vi "DiffDriveTrainSim_GetOutput_Single.vi"(9 "Row":i32, 11 "DiffDriveTrainSim":T1 {"m_Motor"."Jr_KgM2" format="%13.5p"; "m_Motor"."L_H" format="%13.5p"; "m_Motor"."Kt_NMPerAmp" format="%13.5p"; "m_Motor"."KvINV_RadPerSecPerVolt" format="%13.5p"; "m_Motor"."R_Ohms" format="%13.5p"; "m_Motor"."FreeSpeed_RadPerSec" format="%13.5p"; "m_Motor"."FreeCurrent_Amps" format="%13.5p"; "m_Motor"."StallCurrent_Amps" format="%13.5p"; "m_Motor"."StallTorque_NM" format="%13.5p"; "m_Motor"."nominalVoltage_Volts" format="%13.5p"}) -> (3 "Output":dbl)   [LabVIEW 2019, in "Trajectory_Library.lvlib"]
doc: "Get the output \n\nInputs:\n - DiffDriveTraimSim -- Data cluster\n - Row -- The desired row.\n values correspond to:\n 0 = X\n 1 = Y\n 2 = Heading\n 3 = LeftVelocity\n 4 = RightVelocity\n 5 = LeftPosition\n 6 = RightPosition\n\nOutputs:\n - Output -- The output value"
uses:
  Trajectory_Library.lvlib
  TypeDef/LINEAR_SYSTEM.ctl
  <vilib>/Analysis/Matrix/Datatypes/RealMatrix.ctl
  <vilib>/Analysis/Matrix/NI_Matrix.lvlib
  TypeDef/DCMOTOR.CTL
  TypeDef/DIFF_DRIVE_TRAIN_SIM.ctl
panel:
  # "<States, 1>"
  # "<Outputs, 1>"
  # "<Inputs, 1>"
  # "<Outputs, 1>"
  # "<States,States>"
  # "<States,Inputs>"
  # "<Outputs,States>"
  # "<Outputs,Inputs>"
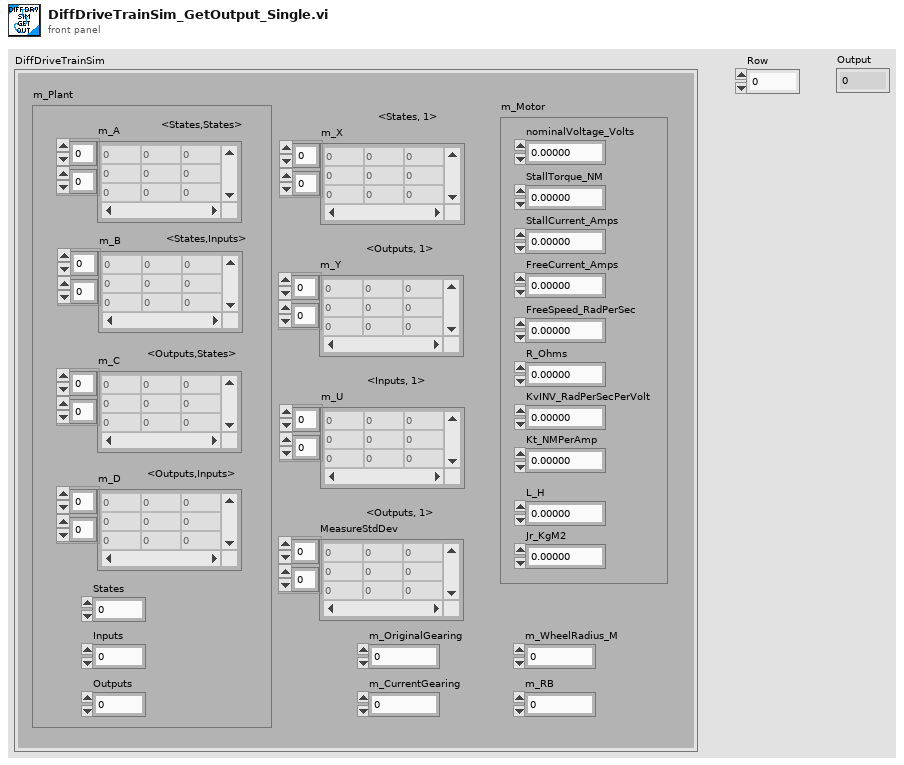
[diagram p1: front panel]
types:
  T1 = typedef "Trajectory_Library.lvlib/DIFF_DRIVE_TRAIN_SIM.ctl" = cluster{"m_Plant":T2, "m_X":T3, "m_Y":T3, "m_U":T3, "MeasureStdDev":T3, "m_Motor":T4, "m_OriginalGearing":dbl, "m_CurrentGearing":dbl, "m_WheelRadius_M":dbl, "m_RB":dbl}
  T2 = typedef "Trajectory_Library.lvlib/LINEAR_SYSTEM.ctl" = cluster{"m_A":T3, "m_B":T3, "m_C":T3, "m_D":T3, "States":i32, "Inputs":i32, "Outputs":i32}
  T3 = typedef "NI_Matrix.lvlib/RealMatrix.ctl" = dbl[][]
  T4 = typedef "Trajectory_Library.lvlib/DCMOTOR.CTL" = cluster{"nominalVoltage_Volts":dbl, "StallTorque_NM":dbl, "StallCurrent_Amps":dbl, "FreeCurrent_Amps":dbl, "FreeSpeed_RadPerSec":dbl, "R_Ohms":dbl, "KvINV_RadPerSecPerVolt":dbl, "Kt_NMPerAmp":dbl, "L_H":dbl, "Jr_KgM2":dbl}
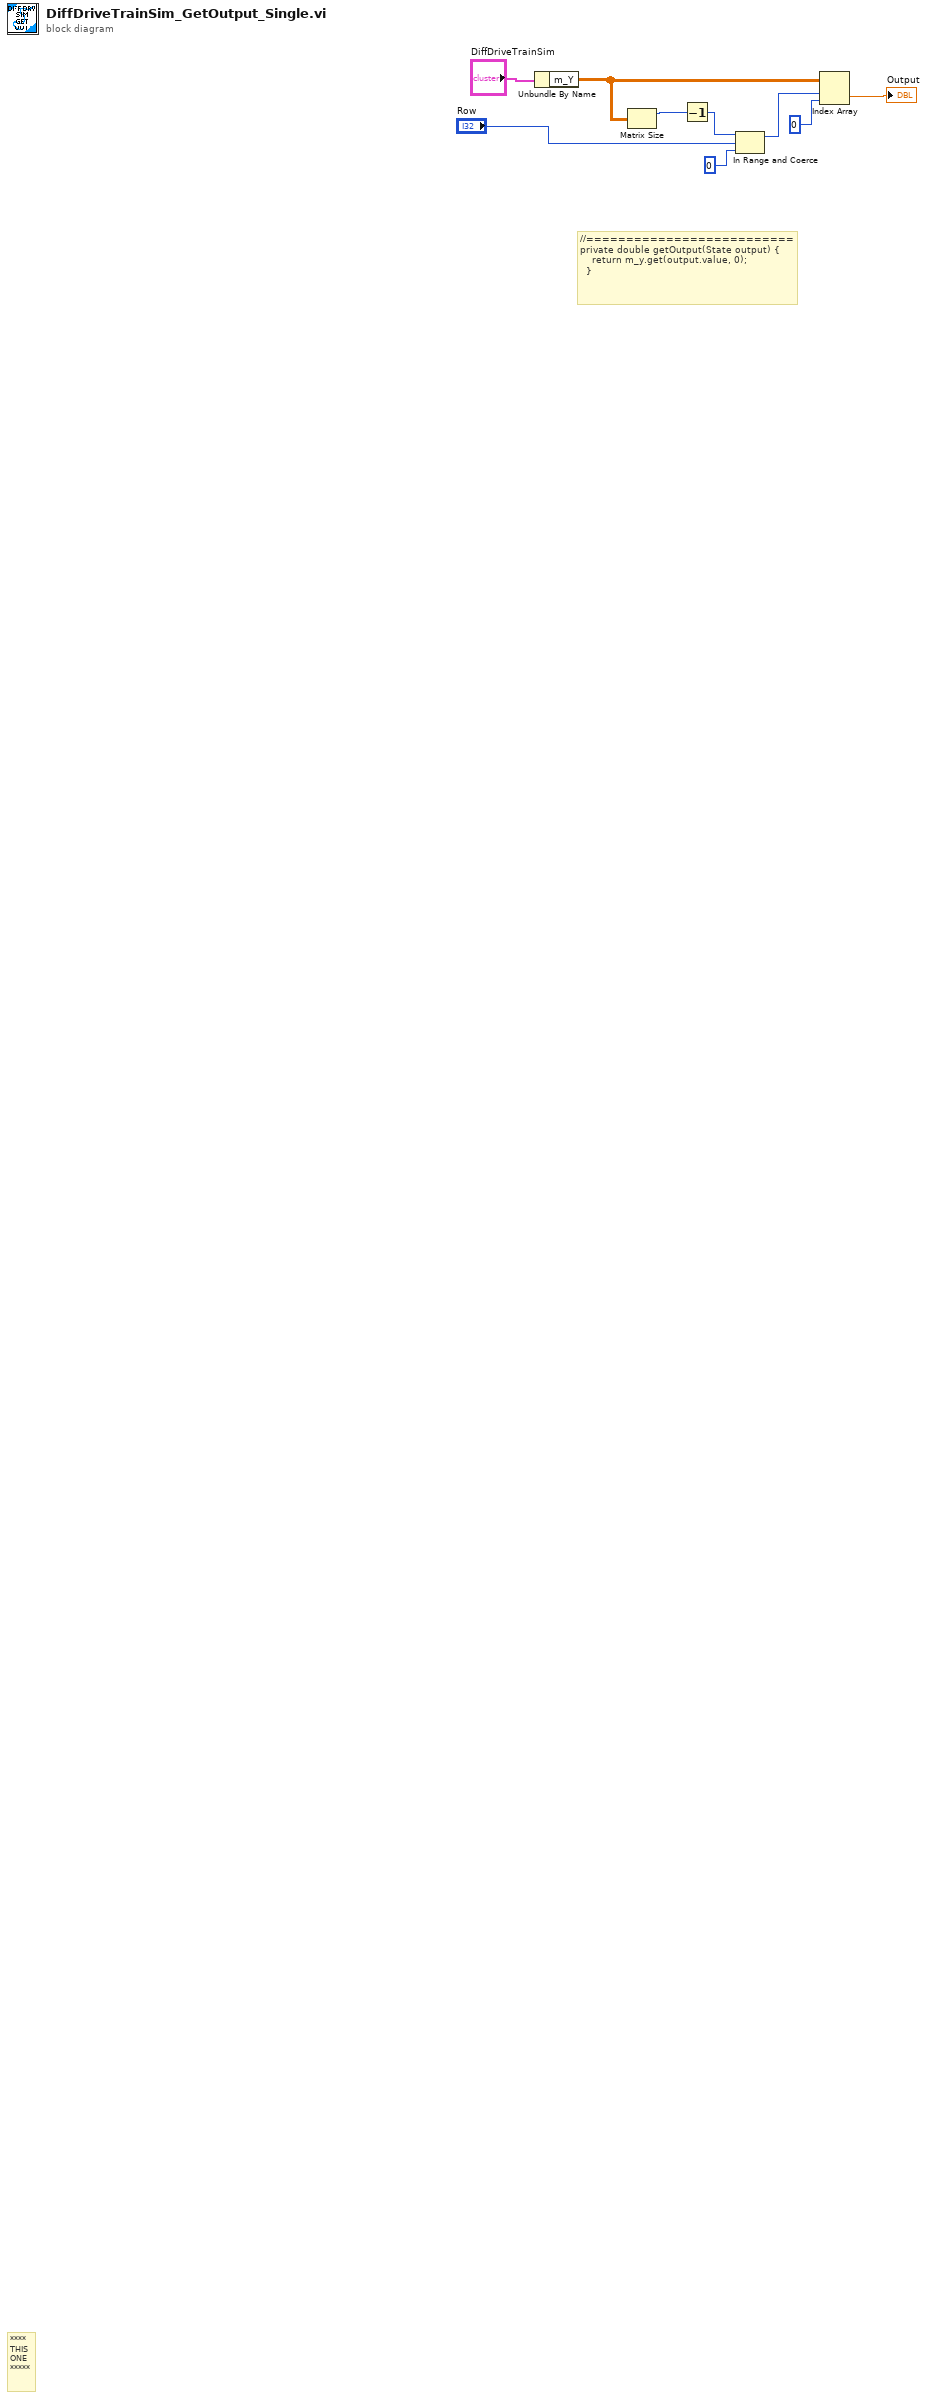
[diagram p0: block diagram]
diagram:
  # "//==========================  \nprivate double getOutput(State output) {\n    return m_y.get(output.value, 0);\n  }"
  # "****\nTHIS\nONE\n*****"
  n1 = Unbundle By Name("DiffDriveTrainSim") -> ("m_Y"=w2:T3)
  n2 = Matrix Size(0:w2) -> (1:w7:i32)  [unwired: 1 out]
  n3 = Decrement(x=w7) -> (x-1=w8:i32)
  n4 = In Range and Coerce(upper limit=w8, x="Row", lower limit=0) -> (coerced(x)=w4:i32)  [unwired: 1 out]
  n5 = Index Array(array=w2, index (row)=w4, index (col)=0) -> (element=→"Output":dbl)
